vi "pco.camera_Simple_Example_IMAQ.vi"() -> ()   [LabVIEW 2020]
uses:
  Camera.lvclass
panel:
  out "rawImage":u16[][](array[numeric])
  out "Image":T1(plugin-control)
  in  "data_format":T2(ring)=enum."Mono16"
  in  "Image Index":u32 max=99
  out "Recorded Images":u32
  in  "Quit":bool
  in  "roiY1":u64=2 min=2 max=1040 step=1
  in  "roiX1":u64=2 min=2 max=1392 step=1
  in  "roiY0":u64=1 min=1 max=1039 step=1
  in  "roiX0":u64=1 min=1 max=1391 step=1
  out "Image Height":u16
  out "Image Width":u16
  in  "dwImgCount":u32=10 caption="Required Number of Images" max=4023
  out "Error":errorcluster {"code" format="%x"}
  # "This example shows a simple recording of an image sequence and the image access afterwards.\nIt is a good starting point for writing own applications.\nBut it will not be fail save, i.e. doesnt react on errors, just handles them forward to the end\n\nUsage:\nSelect your required image count before you start the program.\nOnce started, the camera class will be initialized and images will be recorded automatically.\nWhen acquisition has finished you can address the images and set a certain roi \nTo finish the program click on quit application, this will force fan exit of the camera class"
  # "pco.labview"
  # "Camera Setup"
  # "Recording Control"
  # "Parameters for image readout"
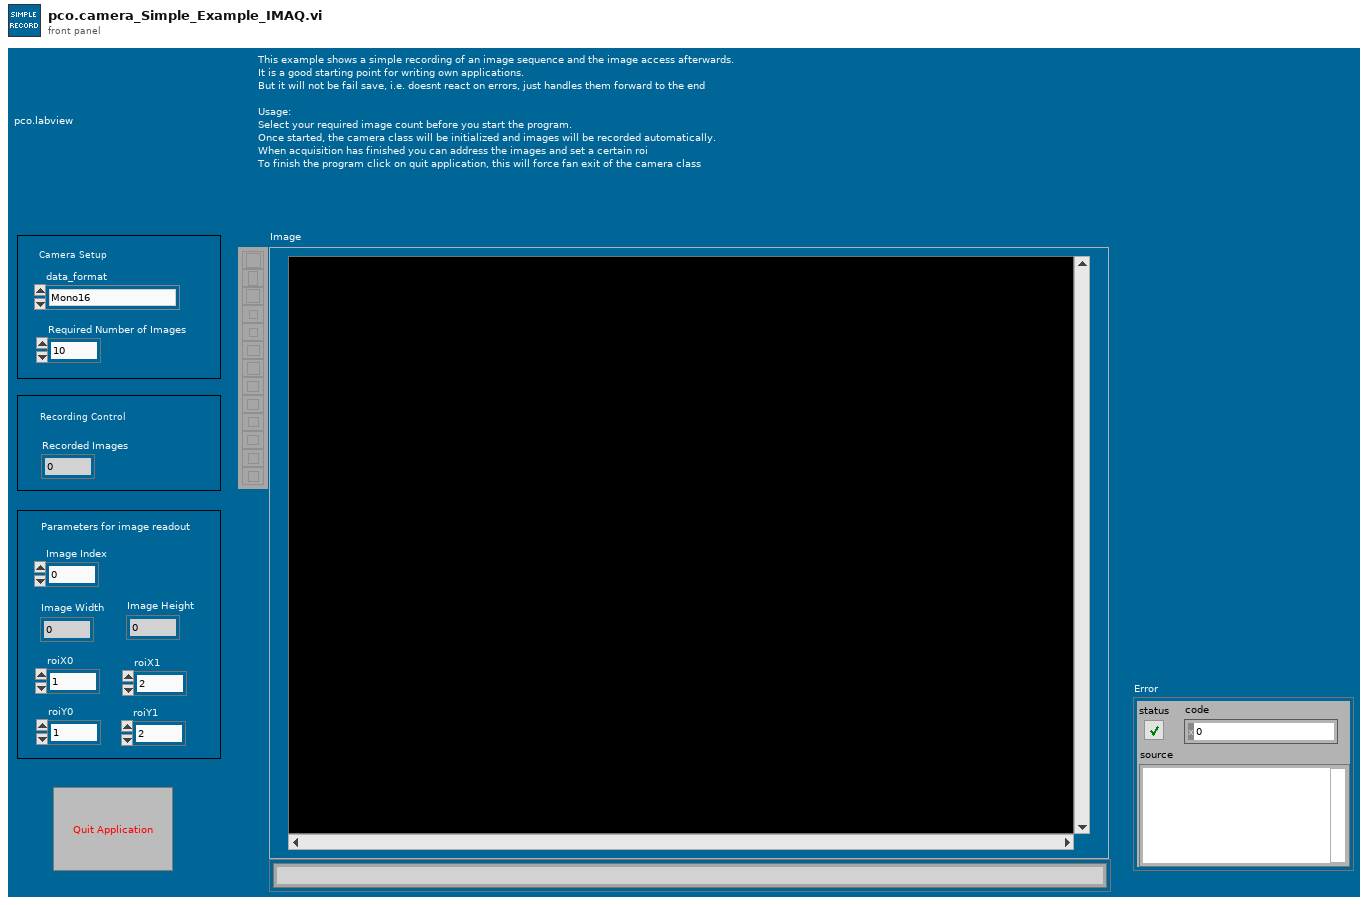
[diagram p1: front panel]
types:
  T1 = typedef "IMAQ Image.ctl" = refnum<image>
  T2 = enum16{"Undefined", "Mono8", "Mono16", "BGRA8", "RGBA8", "BGRA16", "RGBA16", "CompressedMono8"}
  T3 = enum8{"Enabled", "Disabled", "Disabled and Grayed Out"}
  T4 = enum16{"sequence", "sequence non blocking", "ring buffer", "fifo", "sequence_dpcore", "sequence_non_blocking_dpcore", "ring_buffer_dpcore", "fifo_dpcore", "tif", "multitif", "pcoraw", "b16", "dicom", "multidicom"}
  T5 = cluster{"serial":u32, "type":u16, "sub_type":u16, "interface_type":u16, "bit_resolution":u16, "min_exposure_time_s":dbl, "max_exposure_time_s":dbl, "min_exposure_step_s":dbl, "min_delay_time_s":dbl, "max_delay_time_s":dbl, "min_delay_step_s":dbl, "min_width":u64, "min_height":u64, "max_width":u64, "max_height":u64, "roi_step_horz":u64, "roi_step_vert":u64, "roi_symmetric_horz":bool, "roi_symmetric_vert":bool, "has_timestamp_mode":bool, "has_timestamp_mode_ascii_only":bool, "pixelrate_vec":u32[], "has_acquire_mode":bool, "has_ext_acquire_mode":bool, "has_metadata_mode":bool, "has_ram":bool, "binning_horz_vec":u16[], "binning_vert_vec":u16[]}
  T6 = typedef "Image Type" = u32
  T7 = typedef "Camera.lvclass/binning.ctl" = cluster{"vert":u16, "horz":u16}
  T8 = cluster{"exposure_time_s":dbl, "delay_time_s":dbl, "roi":cluster{"x0":u64, "y0":u64, "x1":u64, "y1":u64}, "timestamp_mode":u16, "pixelrate":u32, "trigger_mode":u16, "acquire_mode":u16, "metadata_mode":u16, "noisefilter_mode":u16, "binning":T7}
  T9 = cluster{"Plane 4 (alpha)":u16, "Plane 1 (Red)":u16, "Plane 2 (Green)":u16, "Plane 3 (Blue)":u16}[][]
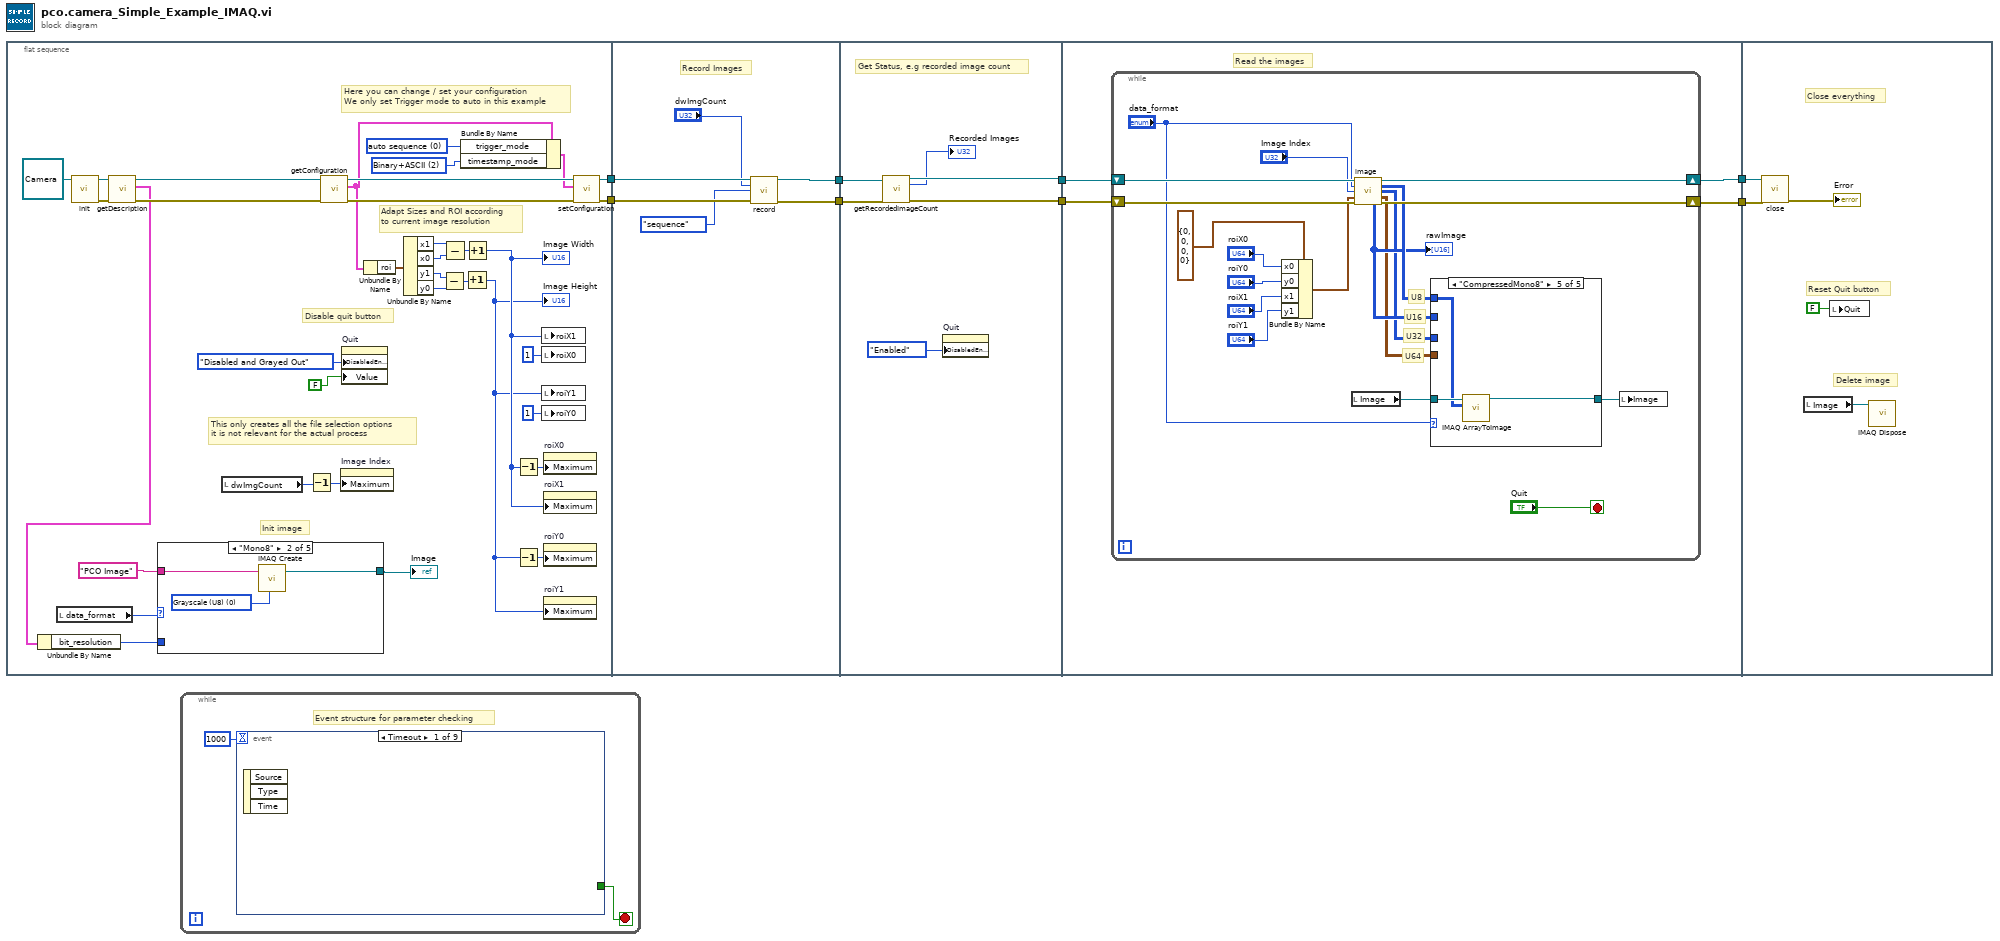
[diagram p0: block diagram]
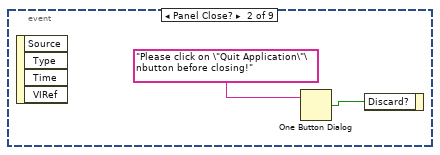
[diagram p2: hidden frame]
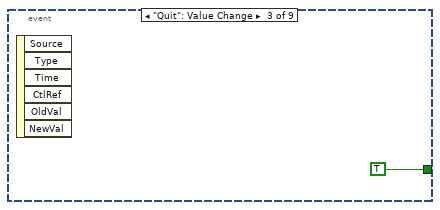
[diagram p3: hidden frame]
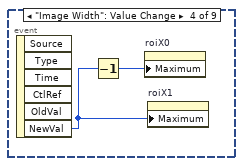
[diagram p4: hidden frame]
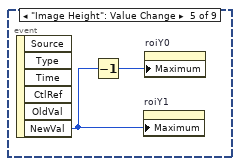
[diagram p5: hidden frame]
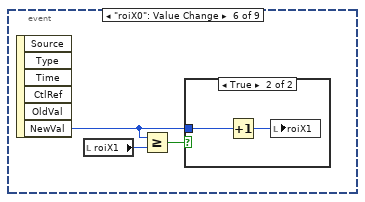
[diagram p6: hidden frame]
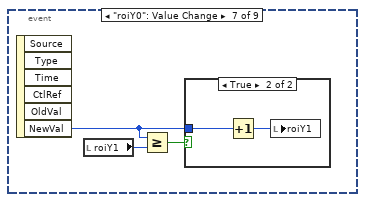
[diagram p8: hidden frame]
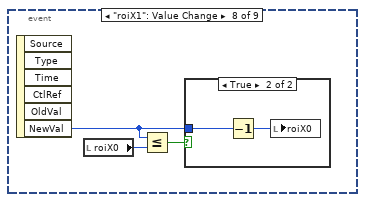
[diagram p10: hidden frame]
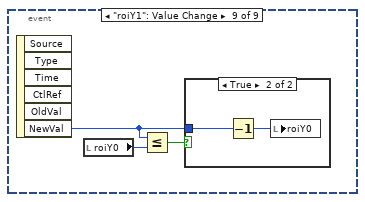
[diagram p12: hidden frame]
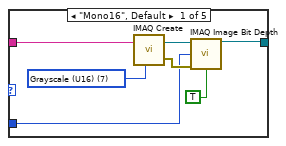
[diagram p14: hidden frame]
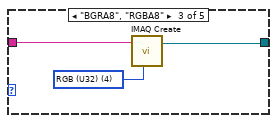
[diagram p15: hidden frame]
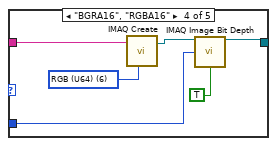
[diagram p16: hidden frame]
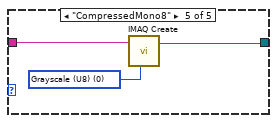
[diagram p17: hidden frame]
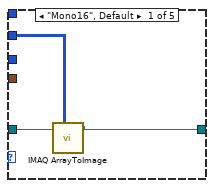
[diagram p18: hidden frame]
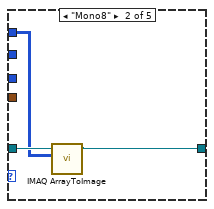
[diagram p19: hidden frame]
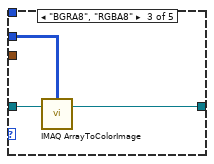
[diagram p20: hidden frame]
diagram:
  n1 = flat-sequence {
    tunnel: [w38] -> w8
    tunnel: [w37] -> w7
    tunnel: w8 -> [w71]
    tunnel: w7 -> [w70]
    tunnel: [w68] -> w6
    tunnel: [w67] -> w5
    tunnel: w6 -> [w77]
    tunnel: w5 -> [w76]
    tunnel: [w75] -> w4
    tunnel: [w74] -> w3
    tunnel: w4 -> [w80]
    tunnel: w3 -> [w81]
    tunnel: [w79] -> w2
    tunnel: [w78] -> w1
    tunnel: w2 -> [w118]
    tunnel: w1 -> [w117]
    frame #0 {
      w22 = u16 2 items=["OFF", "Binary", "Binary+ASCII", "ASCII"] ("TimestampMode")
      w42 = u16 0 items=["auto sequence"=0, "software trigger"=1, "external exposure start & software trigger"=2, "external exposure control"=3, "external synchronized"=4, "fast external exposure control"=5, "external CDS control"=6, "slow external exposure control"=7, "external synchronized HDSDI"=258] ("TriggerMode")
      # "Init image"
      # "This only creates all the file selection options\nit is not relevant for the actual process"
      # "Adapt Sizes and ROI according\nto current image resolution"
      # "Disable quit button"
      # "Here you can change / set your configuration\nWe only set Trigger mode to auto in this example"
      n2 = local read "data_format"() -> (w17:T2)
      n3 = call-dynamic "init.vi"("Camera in"=refnum<class "Camera.lvclass"> refnum ("PCOCamera in")) -> ("Camera out"=w13:refnum<class "Camera.lvclass">, "error out"=w14:errorcluster)  [unwired: 8 in]
      n4 = call-dynamic "getDescription.vi"("error in (no error)"=w14, "Camera in"=w13) -> ("error out"=w11:errorcluster, "description"=w10:T5, "Camera out"=w12:refnum<class "Camera.lvclass">)  [unwired: 7 in]
      n5 = Unbundle By Name(w10) -> ("bit_resolution"=w9:u16)
      n6 = case shown="\"Mono8\"" w17 {
        tunnel: "PCO Image" ("Image Name") -> [w49 w53 w55 w61 w64]
        tunnel: [w45 w51 w54 w58 w63] -> w16
        tunnel: w9 -> [w44 _ _ w57 _]
        frame "Mono16", Default {
          w50 = T6 7 items=["Grayscale (U8)", "Grayscale (I16)", "Grayscale (SGL)", "Complex (CSG)", "RGB (U32)", "HSL (U32)", "RGB (U64)", "Grayscale (U16)"] ("Image Type")
          n7 = call "IMAQ Create"("Image Name"=w49, "Image Type"=w50) -> ("New Image"=w47:T1, "error out"=w46:errorcluster)  [unwired: 3 in]
          n8 = call "IMAQ Image Bit Depth"("Image"=w47, "Bit Depth (0)"=w44, "error in (no error)"=w46, "Get/Set Bit Depth? (Set)"=TRUE) -> ("Image Out"=w45:T1)  [unwired: 9 in, 2 out]
        }
        frame "Mono8" {
          w52 = T6 0 items=["Grayscale (U8)", "Grayscale (I16)", "Grayscale (SGL)", "Complex (CSG)", "RGB (U32)", "HSL (U32)", "RGB (U64)", "Grayscale (U16)"] ("Image Type")
          n9 = call "IMAQ Create"("Image Name"=w53, "Image Type"=w52) -> ("New Image"=w51:T1)  [unwired: 3 in, 1 out]
        }
        frame "BGRA8", "RGBA8" {
          w56 = T6 4 items=["Grayscale (U8)", "Grayscale (I16)", "Grayscale (SGL)", "Complex (CSG)", "RGB (U32)", "HSL (U32)", "RGB (U64)", "Grayscale (U16)"] ("Image Type")
          n10 = call "IMAQ Create"("Image Name"=w55, "Image Type"=w56) -> ("New Image"=w54:T1)  [unwired: 3 in, 1 out]
        }
        frame "BGRA16", "RGBA16" {
          w62 = T6 6 items=["Grayscale (U8)", "Grayscale (I16)", "Grayscale (SGL)", "Complex (CSG)", "RGB (U32)", "HSL (U32)", "RGB (U64)", "Grayscale (U16)"] ("Image Type")
          n11 = call "IMAQ Create"("Image Name"=w61, "Image Type"=w62) -> ("New Image"=w59:T1)  [unwired: 3 in, 1 out]
          n12 = call "IMAQ Image Bit Depth"("Image"=w59, "Bit Depth (0)"=w57, "Get/Set Bit Depth? (Set)"=TRUE) -> ("Image Out"=w58:T1)  [unwired: 10 in, 2 out]
        }
        frame "CompressedMono8" {
          w65 = T6 0 items=["Grayscale (U8)", "Grayscale (I16)", "Grayscale (SGL)", "Complex (CSG)", "RGB (U32)", "HSL (U32)", "RGB (U64)", "Grayscale (U16)"] ("Image Type")
          n13 = call "IMAQ Create"("Image Name"=w64, "Image Type"=w65) -> ("New Image"=w63:T1)  [unwired: 3 in, 1 out]
        }
      }
      "Image" <- w16
      n14 = local read "dwImgCount"() -> (w18:u32)
      n15 = Decrement(x=w18) -> (x-1=w19:u32)
      n16 = call-dynamic "getConfiguration.vi"("error in (no error)"=w11, "Camera in"=w12) -> ("error out"=w40:errorcluster, "configuration"=w32:T8, "Camera out"=w41:refnum<class "Camera.lvclass">)  [unwired: 7 in]
      n17 = property on="Image Index" class="DigNum (strict)"("Maximum"=w19) -> ()  [unwired: 2 in, 2 out]
      n18 = property on="Quit" class="Bool (strict)"("DisabledEnum"=T3."Disabled and Grayed Out" ("Disabled"), "Value"=FALSE ("Stop")) -> ()  [unwired: 2 in, 2 out]
      n19 = Unbundle By Name(w32) -> ("roi"=w31:cluster{"x0":u64, "y0":u64, "x1":u64, "y1":u64})
      n20 = Unbundle By Name(w31) -> ("x1"=w29:u64, "x0"=w30:u64, "y1"=w27:u64, "y0"=w28:u64)
      n21 = Subtract(x=w27, y=w28) -> (x-y=w25:u64)
      n22 = Subtract(x=w29, y=w30) -> (x-y=w26:u64)
      n23 = Bundle By Name(cluster=w32, "trigger_mode"=w42, "timestamp_mode"=w22) -> (w39:T8)
      n24 = Increment(x=w25) -> (x+1=w23:u64)
      "Image Height" <- w23
      n25 = Increment(x=w26) -> (x+1=w24:u64)
      "Image Width" <- w24
      n26 = Decrement(x=w24) -> (x-1=w34:u64)
      n27 = Decrement(x=w23) -> (x-1=w33:u64)
      n28 = local write "roiX1"(w24) -> ()
      n29 = local write "roiX0"(u16 1 ("roiY0")) -> ()
      n30 = local write "roiY1"(w23) -> ()
      n31 = local write "roiY0"(u16 1 ("roiY0")) -> ()
      n32 = property on="roiX0" class="DigNum (strict)"("Maximum"=w34) -> ()  [unwired: 2 in, 2 out]
      n33 = property on="roiX1" class="DigNum (strict)"("Maximum"=w24) -> ()  [unwired: 2 in, 2 out]
      n34 = property on="roiY0" class="DigNum (strict)"("Maximum"=w33) -> ()  [unwired: 2 in, 2 out]
      n35 = property on="roiY1" class="DigNum (strict)"("Maximum"=w23) -> ()  [unwired: 2 in, 2 out]
      n36 = call-dynamic "setConfiguration.vi"("error in (no error)"=w40, "configuration"=w39, "Camera in"=w41) -> ("error out"=w37:errorcluster, "Camera out"=w38:refnum<class "Camera.lvclass">)  [unwired: 7 in]
    }
    frame #1 {
      # "Record Images"
      n37 = call-dynamic "record.vi"("Camera in"=w71, "num_images"="dwImgCount", "record_mode"=T4."sequence", "error in (no error)"=w70) -> ("Camera out"=w68:refnum<class "Camera.lvclass">, "error out"=w67:errorcluster)  [unwired: 10 in]
    }
    frame #2 {
      # "Get Status, e.g recorded image count"
      n38 = call-dynamic "getRecordedImageCount.vi"("Camera in"=w77, "error in (no error)"=w76) -> ("Camera out"=w75:refnum<class "Camera.lvclass">, "recorded_image_count"=→"Recorded Images":u32, "error out"=w74:errorcluster)  [unwired: 11 in]
      n39 = property on="Quit" class="Bool (strict)"("DisabledEnum"=T3."Enabled" ("Disabled")) -> ()  [unwired: 2 in, 2 out]
    }
    frame #3 {
      # "Read the images"
      n40 = while {
        shift-right: [w98] -> w79
        shift-left: w80 -> [w100]
        shift-right: [w93] -> w78
        shift-left: w81 -> [w99]
        stop <- "Quit" stop-if-true
        # "U64"
        # "U32"
        # "U16"
        # "U8"
        n41 = Bundle By Name(cluster=cluster{"x0":u64, "y0":u64, "x1":u64, "y1":u64} {"x0"=0, "y0"=0, "x1"=0, "y1"=0} ("roi"), "x0"="roiX0", "y0"="roiY0", "x1"="roiX1", "y1"="roiY1") -> (w92:cluster{"x0":u64, "y0":u64, "x1":u64, "y1":u64})
        n42 = local read "Image"() -> (w85:T1)
        n43 = call-dynamic "image.vi"("Camera in"=w100, "data_format"="data_format", "image_index"="Image Index", "roi"=w92, "error in (no error)"=w99) -> ("Camera out"=w98:refnum<class "Camera.lvclass">, "image (U8)"=w89:u8[][], "image (U32)"=w87:u32[][], "image (U64)"=w86:T9, "raw_image (U16)"=w88:u16[][], "error out"=w93:errorcluster)  [unwired: 3 in, 2 out]
        "rawImage" <- w88
        n44 = case shown="\"CompressedMono8\"" "data_format" {
          tunnel: w85 -> [w103 w106 w109 w112 w115]
          tunnel: [w101 w104 w108 w110 w114] -> w84
          tunnel: w86 -> [_ _ _ w111 _]
          tunnel: w87 -> [_ _ w107 _ _]
          tunnel: w89 -> [_ w105 _ _ w113]
          tunnel: w88 -> [w102 _ _ _ _]
          frame "Mono16", Default {
            n45 = call "IMAQ ArrayToImage"("Image Pixels (U16)"=w102, "Image"=w103) -> ("Image Out"=w101:T1)  [unwired: 8 in, 1 out]
          }
          frame "Mono8" {
            n46 = call "IMAQ ArrayToImage"("Image Pixels (U8)"=w105, "Image"=w106) -> ("Image Out"=w104:T1)  [unwired: 8 in, 1 out]
          }
          frame "BGRA8", "RGBA8" {
            n47 = call "IMAQ ArrayToColorImage"("Image Pixels (U32)"=w107, "Image"=w109) -> ("Image Out"=w108:T1)  [unwired: 3 in, 1 out]
          }
          frame "BGRA16", "RGBA16" {
            n48 = call "IMAQ ArrayToColorImage"("Image"=w112, "Image Pixels (U64)"=w111) -> ("Image Out"=w110:T1)  [unwired: 3 in, 1 out]
          }
          frame "CompressedMono8" {
            n49 = call "IMAQ ArrayToImage"("Image Pixels (U8)"=w113, "Image"=w115) -> ("Image Out"=w114:T1)  [unwired: 8 in, 1 out]
          }
        }
        n50 = local write "Image"(w84) -> ()
      }
    }
    frame #4 {
      # "Delete image"
      # "Reset Quit button"
      # "Close everything"
      n51 = call-dynamic "close.vi"("error in (no error)"=w117, "Camera in"=w118) -> ("error out"=→"Error":errorcluster)  [unwired: 9 in]
      n52 = local read "Image"() -> (w116:T1)
      n53 = local write "Quit"(FALSE ("Stop")) -> ()
      n54 = call "IMAQ Dispose"("Image"=w116) -> ()  [unwired: 5 in, 1 out]
    }
  }
  n55 = while {
    stop <- w121 stop-if-true
    # "Event structure for parameter checking"
    n56 = event shown="[0] Timeout" {
      selector: _ -> [_ _ _ _ _ _ _ _ _]
      dyn-events: _ -> [_ _ _ _ _ _ _ _ _]
      timeout: 1000 -> [_ _ _ _ _ _ _ _ _]
      tunnel: [_ _ TRUE _ _ _ _ _ _] -> w121
      event Timeout {
        n57 = event-data() -> ()  [unwired: 1 in, 3 out]
      }
      event Panel Close? {
        n58 = event-data() -> ()  [unwired: 1 in, 4 out]
        n59 = One Button Dialog(message="Please click on \"Quit Application\"\nbutton before closing!") -> (true=w123:bool)  [unwired: 1 in]
        n60 = event-data("Discard?"=w123) -> ()  [unwired: 1 in, 1 out]
      }
      event "Quit": Value Change {
        n61 = event-data() -> ()  [unwired: 1 in, 6 out]
      }
      event "Image Width": Value Change {
        n62 = event-data() -> ("NewVal"=w126:u16)  [unwired: 1 in, 5 out]
        n63 = Decrement(x=w126) -> (x-1=w127:u16)
        n64 = property on="roiX0" class="DigNum (strict)"("Maximum"=w127) -> ()  [unwired: 2 in, 2 out]
        n65 = property on="roiX1" class="DigNum (strict)"("Maximum"=w126) -> ()  [unwired: 2 in, 2 out]
      }
      event "Image Height": Value Change {
        n66 = event-data() -> ("NewVal"=w128:u16)  [unwired: 1 in, 5 out]
        n67 = Decrement(x=w128) -> (x-1=w129:u16)
        n68 = property on="roiY1" class="DigNum (strict)"("Maximum"=w128) -> ()  [unwired: 2 in, 2 out]
        n69 = property on="roiY0" class="DigNum (strict)"("Maximum"=w129) -> ()  [unwired: 2 in, 2 out]
      }
      event "roiX0": Value Change {
        n70 = event-data() -> ("NewVal"=w130:u64)  [unwired: 1 in, 5 out]
        n71 = local read "roiX1"() -> (w132:u64)
        n72 = Greater Or Equal?(x=w130, y=w132) -> (x >= y?=w131:bool)
        n73 = case shown="True" w131 {
          tunnel: w130 -> [_ w134]
          frame False {
          }
          frame True {
            n74 = Increment(x=w134) -> (x+1=w133:u64)
            n75 = local write "roiX1"(w133) -> ()
          }
        }
      }
      event "roiY0": Value Change {
        n76 = event-data() -> ("NewVal"=w135:u64)  [unwired: 1 in, 5 out]
        n77 = local read "roiY1"() -> (w137:u64)
        n78 = Greater Or Equal?(x=w135, y=w137) -> (x >= y?=w136:bool)
        n79 = case shown="True" w136 {
          tunnel: w135 -> [_ w139]
          frame False {
          }
          frame True {
            n80 = Increment(x=w139) -> (x+1=w138:u64)
            n81 = local write "roiY1"(w138) -> ()
          }
        }
      }
      event "roiX1": Value Change {
        n82 = event-data() -> ("NewVal"=w140:u64)  [unwired: 1 in, 5 out]
        n83 = local read "roiX0"() -> (w142:u64)
        n84 = Less Or Equal?(x=w140, y=w142) -> (x <= y?=w141:bool)
        n85 = case shown="True" w141 {
          tunnel: w140 -> [_ w144]
          frame False {
          }
          frame True {
            n86 = Decrement(x=w144) -> (x-1=w143:u64)
            n87 = local write "roiX0"(w143) -> ()
          }
        }
      }
      event "roiY1": Value Change {
        n88 = event-data() -> ("NewVal"=w145:u64)  [unwired: 1 in, 5 out]
        n89 = local read "roiY0"() -> (w147:u64)
        n90 = Less Or Equal?(x=w145, y=w147) -> (x <= y?=w146:bool)
        n91 = case shown="True" w146 {
          tunnel: w145 -> [_ w149]
          frame False {
          }
          frame True {
            n92 = Decrement(x=w149) -> (x-1=w148:u64)
            n93 = local write "roiY0"(w148) -> ()
          }
        }
      }
    }
  }
